vi "HumiditySensorVI.vi"() -> ()   [LabVIEW 2018]
panel:
  out "Relative Humidity":dbl
  out "Relative Humidity":dbl(graph)
  in  "stop":bool
  out "Voltage":dynamicdata(graph)
  out "Voltage":dbl
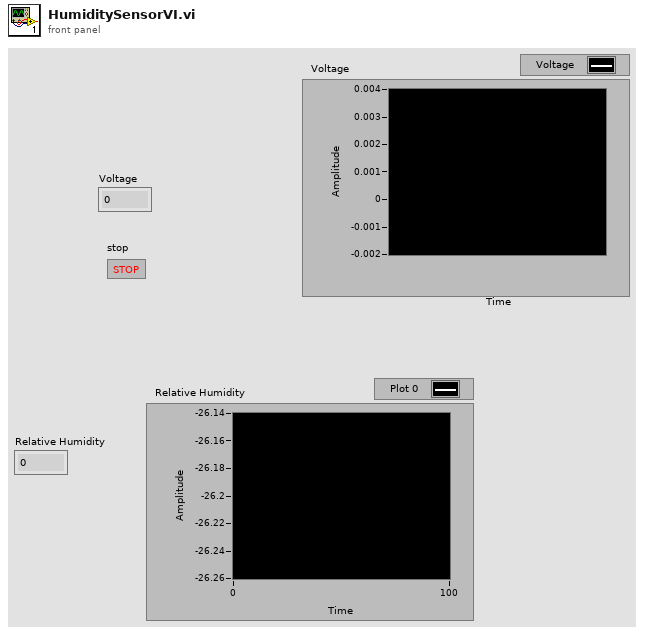
[diagram p1: front panel]
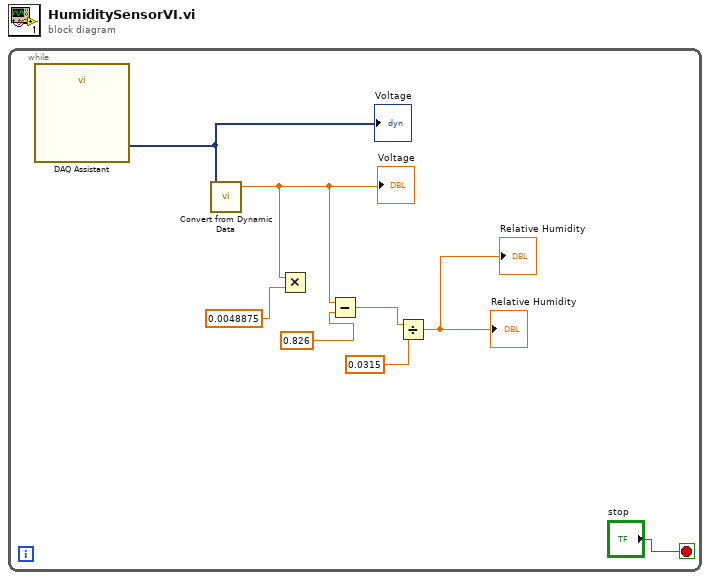
[diagram p0: block diagram]
diagram:
  n1 = while {
    stop <- "stop" stop-if-true
    n2 = call "DAQ Assistant"() -> ("data"=w8:dynamicdata)  [unwired: 16 in, 3 out]
    "Voltage" <- w8
    n3 = call "Convert from Dynamic Data"("Dynamic Data Type"=w8) -> ("Scalar"=w1:dbl)  [unwired: 3 in]
    "Voltage" <- w1
    n4 = Multiply(x=w1, y=0.0048875) -> ()  [unwired: 1 out]
    n5 = Subtract(x=w1, y=0.826) -> (x-y=w4:dbl)
    n6 = Divide(x=w4, y=0.0315) -> (x/y=→"Relative Humidity" →"Relative Humidity":dbl)
  }
